vi "Reset Car.vi"(8 "error in (no error)":errorcluster, 11 "FormulaG API in":refnum<class "FormulaG API.lvclass">) -> (0 "error out":errorcluster, 3 "FormulaG API out":refnum<class "FormulaG API.lvclass">)   [LabVIEW 2020, in "FormulaG.lvlib" / "FormulaG API.lvclass"]
uses:
  FormulaG API.lvclass
  Command.ctl
  FormulaG API.lvclass/FormulaG API.ctl
  <vilib>/IlluminatedG/IG GodotServer/GodotLV/GodotServer/GodotServer.lvclass
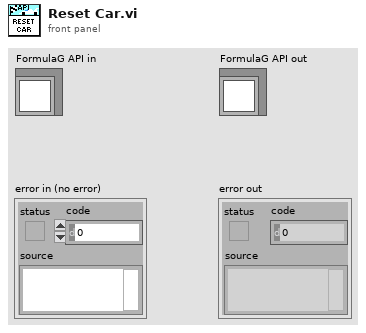
[diagram p1: front panel]
types:
  T1 = typedef "FormulaG.lvlib/FormulaG API.lvclass/Command.ctl" = enum8{"None", "Reset Car", "Request State", "Control Car", "Request Info", "Set Options", "Set Camera", "Set Pause", "Request Time"}
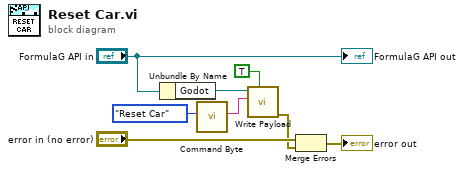
[diagram p0: block diagram]
diagram:
  n1 = Unbundle By Name("FormulaG API in") -> ("Godot"=w6:refnum<class "GodotServer.lvclass">)
  n2 = call "Command Byte.vi"("Command"=Command."Reset Car") -> ("Command Byte"=w5:string)  [unwired: 10 in]
  n3 = call <vilib>:"Write Payload.vi"("Binary (F = Text)"=TRUE, "Payload"=w5, "GodotServer in"=w6) -> ("error out"=w2:errorcluster)  [unwired: 7 in, 1 out]
  n4 = Merge Errors("error in (no error)", w2) -> (→"error out":errorcluster)
  "FormulaG API out" <- "FormulaG API in"
